vi "DBUpdateCopyItem.vi"(8 "error in (no error)":errorcluster, 9 "message value":variant, 11 "ProcessState in":T1) -> (0 "error out":errorcluster, 3 "ProcessState out":T1)   [LabVIEW 2015, in "FileHandler.lvlib"]
uses:
  FileHandler.lvlib
  controls/ProcessState.ctl
  <vilib>/drjdpowell/SQLite Library/SQL Connection/Connection.lvclass
  <vilib>/drjdpowell/SQLite Library/SQL Statement/SQL Statement.lvclass/SQL Statement.ctl
  <vilib>/drjdpowell/SQLite Library/SQL Statement/Bind Path.vi
  <vilib>/drjdpowell/SQLite Library/SQL Statement/Bind Text.vi
  <vilib>/drjdpowell/SQLite Library/SQL Statement/Bind Null.vi
  <vilib>/AdvancedString/Path To Command Line String.vi
  <vilib>/drjdpowell/SQLite Library/SQL Statement/Error Message.vi
  <vilib>/drjdpowell/SQLite Library/SQL Statement/SQL Statement.lvclass
  DBToolkit/DBToolkit.lvlib
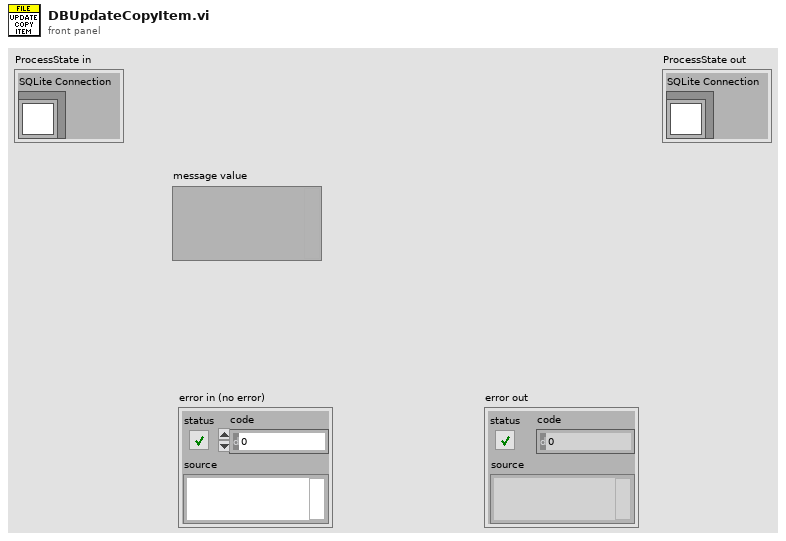
[diagram p1: front panel]
types:
  T1 = typedef "FileHandler.lvlib/ProcessState.ctl" = cluster{"SQLite Connection":refnum<class "Connection.lvclass">}
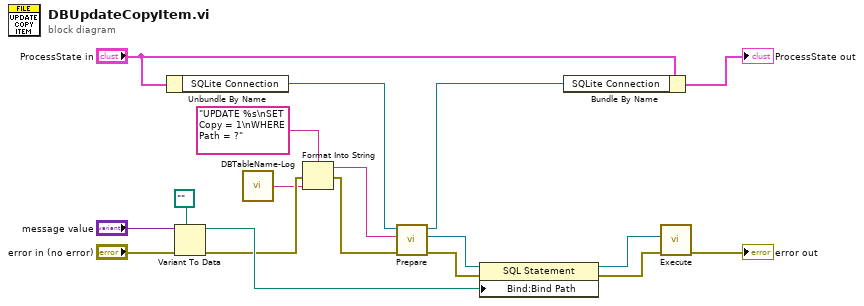
[diagram p0: block diagram]
diagram:
  n1 = Unbundle By Name("ProcessState in") -> ("SQLite Connection"=w7:refnum<class "Connection.lvclass">)
  n2 = Variant To Data(error in="error in (no error)", type=path "", Variant="message value") -> (data=w10:path, error out=w2:errorcluster)
  n3 = call "DBTableName-Log.vi"() -> ("DB Table Name"=w1:string)  [unwired: 5 in]
  n4 = Format Into String(format string="UPDATE %s\nSET Copy = 1\nWHERE Path = ?", error in=w2, w1) -> (resulting string=w4:string, error out=w3:errorcluster)  [unwired: 1 in]
  n5 = call <vilib>:"Prepare.vi"("error in (no error)"=w3, "SQL"=w4, "SQLite Connection in"=w7) -> ("error out"=w8:errorcluster, "SQL Statement out"=w9:refnum<class "SQL Statement.lvclass">, "SQLite Connection out"=w6:refnum<class "Connection.lvclass">)  [unwired: 4 in, 2 out]
  n6 = property class="SQL Statement"(reference=w9, error in=w8, "Bind:Bind Path"=w10) -> (reference out=w14:refnum<class "SQL Statement.lvclass">, error out=w13:errorcluster)
  n7 = Bundle By Name(cluster="ProcessState in", "SQLite Connection"=w6) -> (→"ProcessState out":T1)
  n8 = call "Execute.vi"("error in (no error)"=w13, "SQL Statement in"=w14) -> ("error out"=→"error out":errorcluster)  [unwired: 9 in]
